vi "Read Bottom.vi"(8 "error in (no error)":errorcluster, 11 "Image Assertion in":refnum<class "Image Assertion.lvclass">) -> (0 "error out":errorcluster, 2 "Bottom":i16, 3 "Image Assertion out":refnum<class "Image Assertion.lvclass">)   [LabVIEW 2020, in "MacroAssert.lvlib" / "Image Assertion.lvclass"]
uses:
  Image Assertion.lvclass
  Image Assertion.lvclass/Image Assertion.ctl
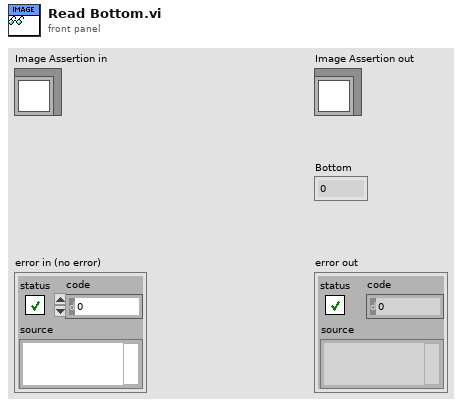
[diagram p1: front panel]
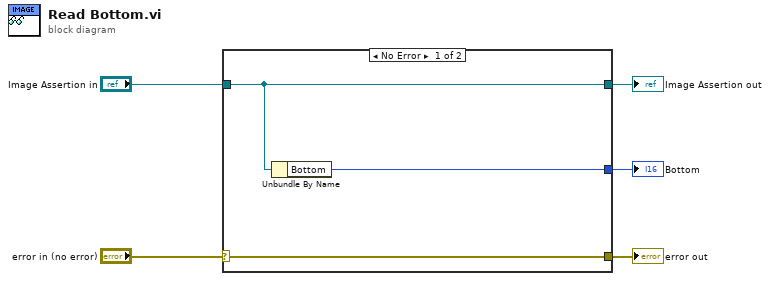
[diagram p0: block diagram]
diagram:
  n1 = case shown="No Error" "error in (no error)" {
    selector: "error in (no error)" -> [w8 w9]
    tunnel: [w8 w9] -> w4
    tunnel: [w7 w10] -> w2
    tunnel: "Image Assertion in" -> [w7 w10]
    tunnel: [w6 _] -> w1
    frame No Error {
      n2 = Unbundle By Name(w7) -> ("Bottom"=w6:i16)
    }
    frame Error {
    }
  }
  "error out" <- w4
  "Image Assertion out" <- w2
  "Bottom" <- w1
